vi "electrical measurements.vi"() -> ()   [LabVIEW 2011]
doc: "This example illustrates how to use autosetup and acquire multiple waveforms from several channels using the following steps:\n\n1. Specify a valid VISA session. \n2. Specify Channel A. \n3. Specify Channel B.\n4. Specify a time-out value for reading waveform.\n5. Run the VI. The graph displays waveforms you acquire."
uses:
  <instrlib>/Tektronix DPO MSO 2000 4000 Series/Public/Configure/Configure Trigger (Edge).vi
  <instrlib>/Tektronix DPO MSO 2000 4000 Series/Public/Data/Read (Multiple Waveforms).vi
  <instrlib>/Tektronix DPO MSO 2000 4000 Series/Tektronix DPO MSO 2000 4000 Series.lvlib
panel:
  in  "Vertical Coupling (1: DC)":u16(ring)=1 items=["AC", "DC", "Ground"]
  in  "Vertical Coupling (1: DC)":u16(ring)=1 items=["AC", "DC", "Ground"]
  in  "Maximum Time (20000ms)":u32=20000
  in  "Current (2: Channel 3)":u16(ring)=1 items=["Channel 1", "Channel 2", "Channel 3", "Channel 4", "Math", "Reference 1", "Reference 2", "Reference 3", "Reference 4"]
  in  "Voltae (0: Channel 1)":u16(ring) items=["Channel 1", "Channel 2", "Channel 3", "Channel 4", "Math", "Reference 1", "Reference 2", "Reference 3", "Reference 4"]
  in  "VISA Resource Name":refnum<visa-resource-name>
  out "Waveform Graph":waveform(dbl)[](graph)
  # "(c) 2006 - 2012. National Instruments Corporation. ALL RIGHTS RESERVED."
  # "High Voltage Probe"
  # "Current probe"
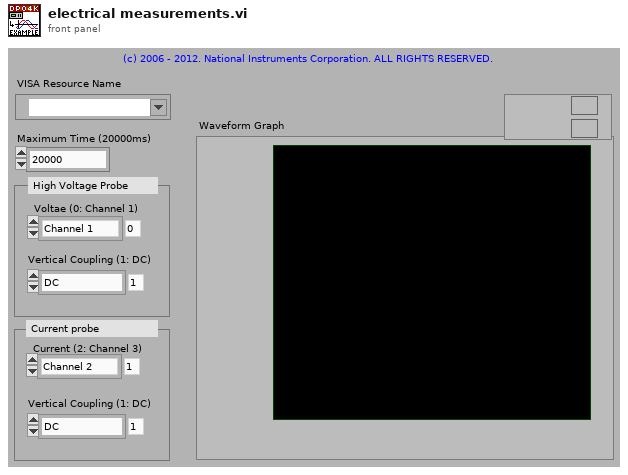
[diagram p1: front panel]
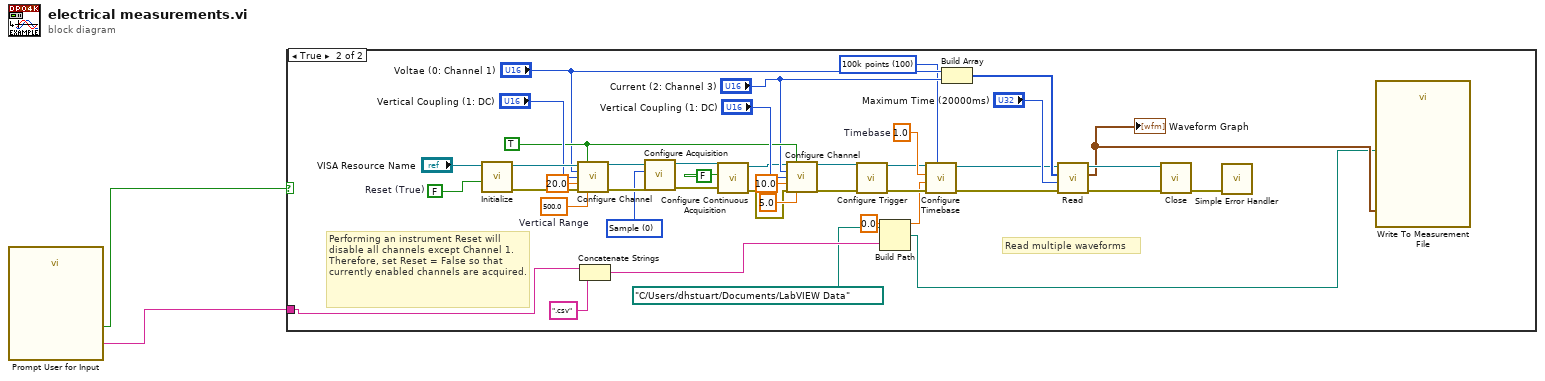
[diagram p0: block diagram]
diagram:
  n1 = call "Prompt User for Input"() -> ("file_name"=w1:string, "OK"=w2:bool)  [unwired: 17 in, 1 out]
  n2 = case shown="True" w2 {
    tunnel: w1 -> [_ w20]
    frame False {
    }
    frame True {
      w3 = u16 0 items=["Sample", "Peak Detect", "Hi Res", "Envelope", "Average"] ("Acquisition Type (0: Sample)")
      w21 = u32 100 items=["1000 points"=1, "10k points"=10, "100k points"=100, "1M points"=1000, "5M points"=5000, "10M points"=10000] ("Record Length (10: 10k points)")
      w30 = 1.0  # Timebase
      w25 = 500.0  # Vertical Range
      w29 = TRUE ("Enable Channel (T: Enable)")
      w37 = FALSE  # Reset (True)
      # "Performing an instrument Reset will disable all channels except Channel 1. Therefore, set Reset = False so that currently enabled channels are acquired."
      # "Read multiple waveforms"
      n3 = call <instrlib>:"Initialize.vi"("Reset (True)"=w37, "VISA resource name"="VISA Resource Name") -> ("error out"=w35:errorcluster, "VISA resource name out"=w36:refnum<visa-resource-name>)  [unwired: 8 in]
      n4 = call <instrlib>:"Configure Channel.vi"("VISA resource name"=w36, "Enable Channel (T: Enable)"=w29, "Channel (0: Channel 1)"="Voltae (0: Channel 1)", "Vertical Coupling (1: DC)"="Vertical Coupling (1: DC)", "Probe Attenuation (1)"=20.0, "error in (no error)"=w35, "Vertical Range (10.0 V)"=w25) -> ("VISA resource name out"=w7:refnum<visa-resource-name>, "error out"=w5:errorcluster)  [unwired: 7 in]
      n5 = Concatenate Strings(w20, ".csv" ("string")) -> (w18:string)
      n6 = call <instrlib>:"Configure Acquisition.vi"("error in (no error)"=w5, "Acquisition Type (0: Sample)"=w3, "VISA resource name"=w7) -> ("error out"=w4:errorcluster, "VISA resource name out"=w6:refnum<visa-resource-name>)  [unwired: 7 in]
      n7 = call <instrlib>:"Configure Continuous Acquisition.vi"("error in (no error)"=w4, "Enable Continuous Acquisition Mode (T: Enable)"=FALSE, "VISA resource name"=w6) -> ("error out"=w9:errorcluster, "VISA resource name out"=w10:refnum<visa-resource-name>)  [unwired: 7 in]
      n8 = call <instrlib>:"Configure Channel.vi"("VISA resource name"=w10, "Enable Channel (T: Enable)"=w29, "Channel (0: Channel 1)"="Current (2: Channel 3)", "Vertical Coupling (1: DC)"="Vertical Coupling (1: DC)", "Probe Attenuation (1)"=10.0, "error in (no error)"=w9, "Vertical Range (10.0 V)"=5.0) -> ("VISA resource name out"=w15:refnum<visa-resource-name>, "error out"=w12:errorcluster)  [unwired: 7 in]
      n9 = call-poly <instrlib>:"Configure Trigger.vi"("VISA resource name"=w15, "error in (no error)"=w12) -> ("VISA resource name out"=w14:refnum<visa-resource-name>, "error out"=w13:errorcluster)  [unwired: 12 in]
      n10 = Build Path(base path=path "C:/Users/dhstuart/Documents/LabVIEW Data", name or relative path=w18) -> (appended path=w16:path)
      n11 = call <instrlib>:"Configure Timebase.vi"("Record Length (10: 10k points)"=w21, "error in (no error)"=w13, "Position (10 %)"=0.0, "Timebase (0.0005 s)"=w30, "VISA resource name"=w14) -> ("error out"=w31:errorcluster, "VISA resource name out"=w32:refnum<visa-resource-name>)  [unwired: 5 in]
      n12 = Build Array("Voltae (0: Channel 1)", "Current (2: Channel 3)") -> (w42:u16[])
      n13 = call-poly <instrlib>:"Read.vi"("error in (no error)"=w31, "Maximum Time (10000ms)"="Maximum Time (20000ms)", "Channels"=w42, "VISA resource name"=w32) -> ("error out"=w40:errorcluster, "Waveform Data"=w26:waveform(dbl)[], "VISA resource name out"=w41:refnum<visa-resource-name>)  [unwired: 5 in]
      "Waveform Graph" <- w26
      n14 = call <instrlib>:"Close.vi"("error in (no error)"=w40, "VISA resource name"=w41) -> ("error out"=w39:errorcluster)  [unwired: 9 in]
      n15 = call <vilib>:"Simple Error Handler.vi"("error in (no error)"=w39) -> ()  [unwired: 4 in, 5 out]
      n16 = call "Write To Measurement File"("Signals"=w26, "Filename"=w16) -> ()  [unwired: 15 in, 3 out]
    }
  }
